vi "MGI Save & Restore Settings.vi"(6 "Section Name (\"Settings\")":string="Settings", 7 "Allow Restore in Development Environment (F)":bool, 8 "Error In":errorcluster, 9 "Command (Restore)":T6, 10 "Path":path, 11 "VI Reference In (Caller)":refnum<vi>) -> (0 "Error Out":errorcluster, 3 "VI Reference Out":refnum<vi>)   [LabVIEW 2016]
doc: "Saves or Restores the settings associated with a VI, including panel bounds, listbox column widths, and graph/chart plots. The settings are saved in an ini file at the specified path. For table style controls, only the columns with headers are saved.\n\nAuthored by Shawn Walpole\nsupport@mooregoodideas.com\nwww.mooregoodideas.com\n\nCopyright (c) 2010, Moore Good Ideas, Inc.\n\nAll rights reserved.\n\nRedistribution and use in source and binary forms, with or without modification, are permitted provided that the following conditions are met:\n\n * Redistributions of source code must retain the above copyright notice, this list of conditions and the following disclaimer.\n * Redistributions in binary form must reproduce the above copyright notice, this list of conditions and the following disclaimer in the documentation and/or other materials provided with the distribution.\n * Neither the name of Moore Good Ideas, Inc. nor the names of its contributors may be used to endorse or promote products derived from this software without specific prior written permission.\n\nTHIS SOFTWARE IS PROVIDED BY THE COPYRIGHT HOLDERS AND CONTRIBUTORS \"AS IS\" AND ANY EXPRESS OR IMPLIED WARRANTIES, INCLUDING, BUT NOT LIMITED TO, THE IMPLIED WARRANTIES OF MERCHANTABILITY AND FITNESS FOR A PARTICULAR PURPOSE ARE DISCLAIMED. IN NO EVENT SHALL THE COPYRIGHT OWNER OR CONTRIBUTORS BE LIABLE FOR ANY DIRECT, INDIRECT, INCIDENTAL, SPECIAL, EXEMPLARY, OR CONSEQUENTIAL DAMAGES (INCLUDING, BUT NOT LIMITED TO, PROCUREMENT OF SUBSTITUTE GOODS OR SERVICES; LOSS OF USE, DATA, OR PROFITS; OR BUSINESS INTERRUPTION) HOWEVER CAUSED AND ON ANY THEORY OF LIABILITY, WHETHER IN CONTRACT, STRICT LIABILITY, OR TORT (INCLUDING NEGLIGENCE OR OTHERWISE) ARISING IN ANY WAY OUT OF THE USE OF THIS SOFTWARE, EVEN IF ADVISED OF THE POSSIBILITY OF SUCH DAMAGE."
uses:
  <userlib>/_MGI/Application Control/MGI Save & Restore Settings/MGI SRS Command Enum.ctl
  <userlib>/_MGI/Application Control/MGI Save & Restore Settings/MGI SRS Graph Setting Cluster.ctl
  <userlib>/_MGI/Application Control/MGI Save & Restore Settings/MGI SRS Graph Plot Cluster.ctl
  <userlib>/_MGI/Application Control/MGI Save & Restore Settings/MGI SRS Graph Cursor Cluster.ctl
  <userlib>/_MGI/Application Control/MGI Save & Restore Settings/MGI SRS MCLB Setting Cluster.ctl
  <userlib>/_MGI/Application Control/MGI Save Restore Settings/Save Restore Settings.lvclass
  <userlib>/_MGI/Application Control/MGI VI Reference/MGI Caller's VI Reference.vi
panel:
  in  "Save Restore Settings in":refnum<class "Save Restore Settings.lvclass">
  in  "Empty":cluster{string, refnum<vi>}[](array[cluster])
  in  "Graph":T1
  in  "MCLB":T4
  in  "Graph":T1
  in  "MCLB":T4
  in  "Empty":cluster{string, refnum<vi>}[](array[cluster])
  in  "Settings":T5
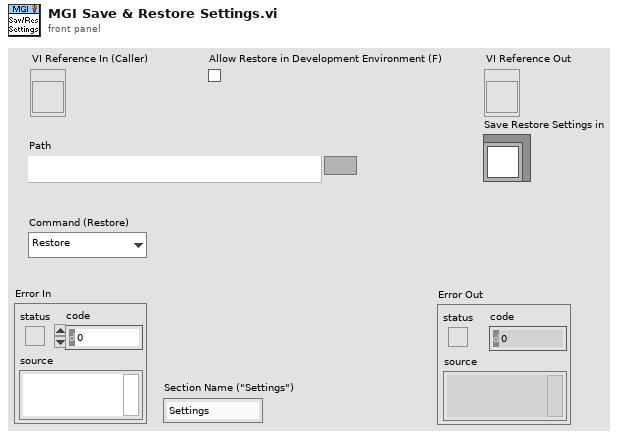
[diagram p1: front panel]
types:
  T1 = typedef "MGI SRS Graph Setting Cluster.ctl" = cluster{"Plot":T2[], "Cursors":T3[], "Cursor Legend?":bool, "Plot Legend?":bool}
  T2 = typedef "MGI SRS Graph Plot Cluster.ctl" = cluster{"Plot Name":string, "Plot Color":u32, "Plot Interpolation":u8, "Point Style":u8, "Line Style":u8, "Fill/Pt. Color":u32, "Line Width":u8, "Bar Plot Style":u8, "Fill To":i16, "XScaleIdx":u32, "YScaleIdx":u32, "Visible?":bool, "Plot Info":cluster{"Plot Color":u32, "Plot Interpolation":u8, "Point Style":u8, "Line Style":u8, "Fill/Pt. Color":u32, "Line Width":u8, "Bar Plot Style":u8, "Fill To":i16}, "Label Style":u8, "Transition Type":u8, "TransitionLocation":u8, "DigitalLineStyle":u8}
  T3 = typedef "MGI SRS Graph Cursor Cluster.ctl" = cluster{"Cursor Name":string, "Cursor Color":u32, "Cursor Style":u8, "Cursor Point Style":u8, "Cursor Name Visible":bool, "Allow Drag":bool, "Cursor Plot":i32, "Cursor Index":i32, "Cursor Position":cluster{"Cursor X":dbl, "Cursor Y":dbl}, "Cursor X":dbl, "Cursor Y":dbl, "Visible":bool, "LineStyle":u8, "LineWidth":u8, "CursorMode":u32, "XScale":u32, "YScale":u32, "WatchPlots":i32[], "WatchAllPlots":bool, "PlotArea":i32, "Label Offset":cluster{"X":dbl, "Y":dbl}}
  T4 = typedef "MGI SRS MCLB Setting Cluster.ctl" = cluster{"Col Widths":i32[]}
  T5 = cluster{"PanelBnds":cluster{"Left":i16, "Top":i16, "Right":i16, "Bottom":i16}, "Splitter Pos":i32[], "Graph Names":string[], "Graph Settings":T1[], "MCLB or Table Names":string[], "MCLB Info":T4[]}
  T6 = typedef "MGI SRS Command Enum.ctl" = enum16{"Restore", "Save"}
  T7 = cluster{"Left":i16, "Top":i16, "Right":i16, "Bottom":i16}
  T8 = typedef "LVRectTypeDef.ctl" = cluster{"Left":i16, "Top":i16, "Right":i16, "Bottom":i16}
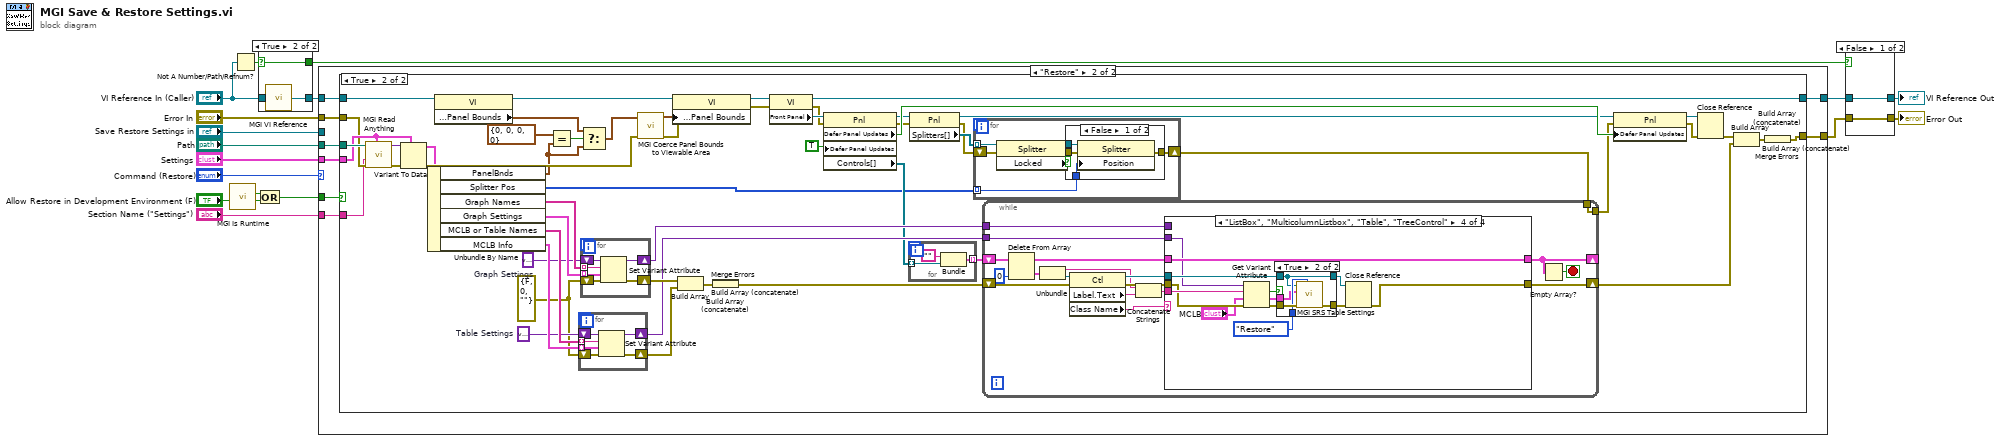
[diagram p0: block diagram]
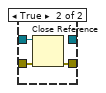
[diagram p2: hidden frame]
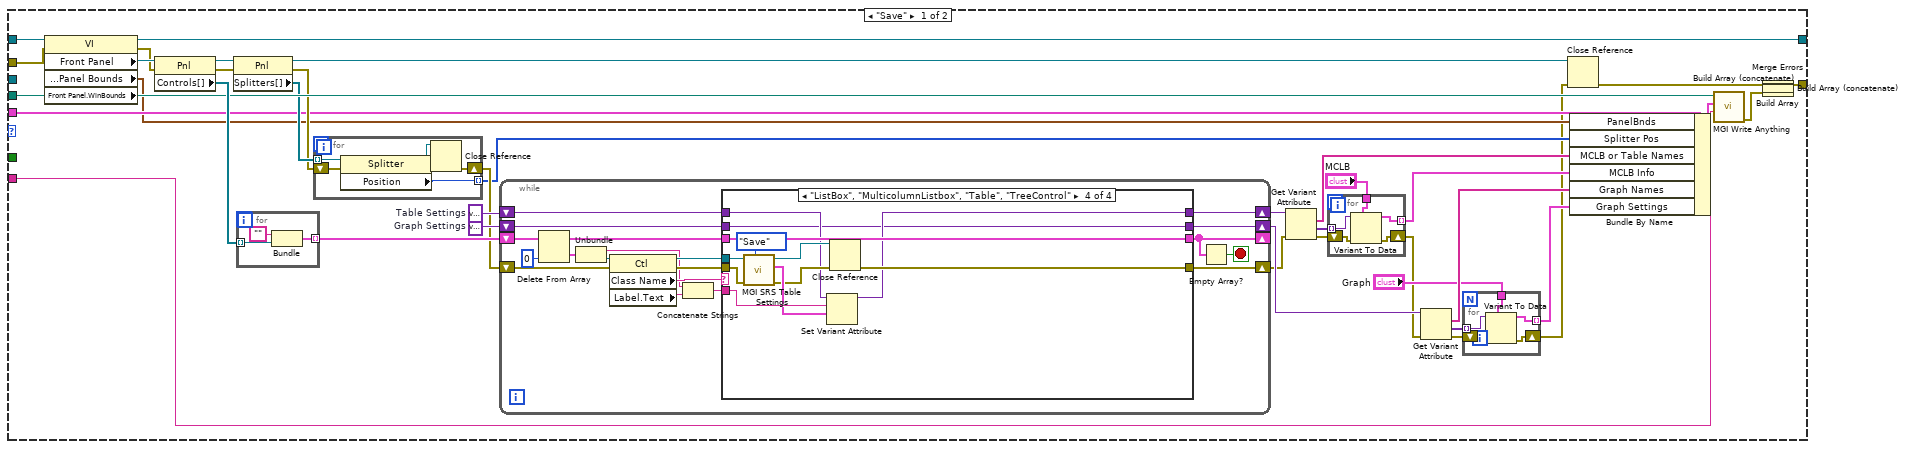
[diagram p3: hidden frame]
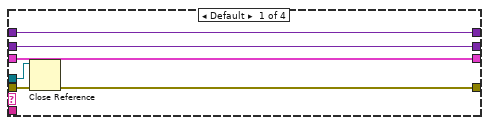
[diagram p4: hidden frame]
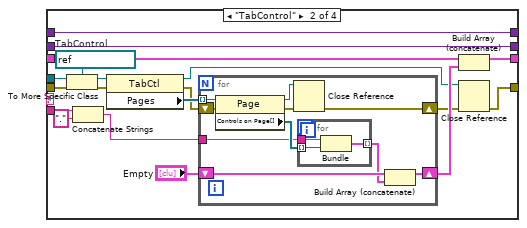
[diagram p5: hidden frame]
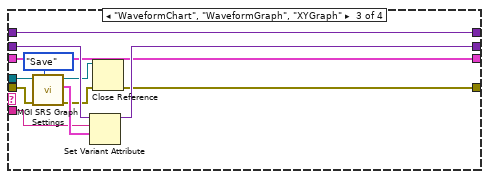
[diagram p6: hidden frame]
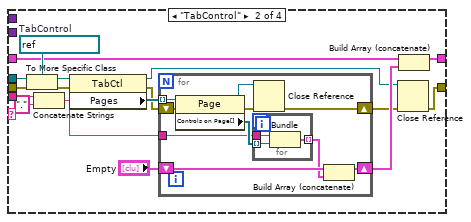
[diagram p10: hidden frame]
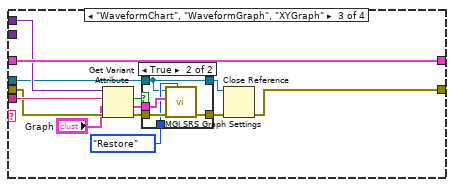
[diagram p11: hidden frame]
diagram:
  n1 = call <userlib>:"MGI Is Runtime.vi"() -> ("Run Time System?"=w4:bool)  [unwired: 7 in]
  n2 = Not A Number/Path/Refnum?(number/path/refnum="VI Reference In (Caller)") -> (NaN/Path/Refnum?=w7:bool)
  n3 = case shown="True" w7 {
    selector: w7 -> [_ w19]
    tunnel: [w18 w20] -> w13
    tunnel: "VI Reference In (Caller)" -> [w18 _]
    tunnel: [_ w19] -> w14
    frame False {
    }
    frame True {
      n4 = call-poly <userlib>:"MGI VI Reference.vi"() -> ("Caller's VI Reference"=w20:refnum<vi>)  [unwired: 1 in]
    }
  }
  n5 = Compound Arithmetic op=OR(w4, "Allow Restore in Development Environment (F)") -> (w3:bool)
  n6 = case shown="\"Restore\"" "Command (Restore)" {
    tunnel: "Path" -> [w43 w167]
    tunnel: [w54 w168] -> w15
    tunnel: "Settings" -> [w32 w166]
    tunnel: w13 -> [w42 w165]
    tunnel: "Error In" -> [w36 w164]
    tunnel: [w25 w163] -> w8
    tunnel: w3 -> [_ w162]
    tunnel: "Section Name (\"Settings\")" -> [w21 w161]
    tunnel: "Save Restore Settings in" -> [_ _]
    frame "Save" {
      w58 = variant  # Graph Settings
      w59 = variant  # Table Settings
      n7 = property class="VI" props=["Front Panel", "Front Panel Window:Panel Bounds", "Front Panel.WinBounds"](reference=w42, error in=w36) -> (reference out=w54:refnum<vi>, error out=w61:errorcluster, "Front Panel"=w62:refnum<vi>, "Front Panel Window:Panel Bounds"=w31:T8)  [unwired: 1 out]
      n8 = property class="Pnl"(reference=w62, error in=w61) -> (reference out=w41:refnum<vi>, error out=w39:errorcluster, "Controls[]"=w60:refnum<vi>[])
      n9 = property class="Pnl"(reference=w41, error in=w39) -> (reference out=w40:refnum<vi>, error out=w37:errorcluster, "Splitters[]"=w38:refnum<vi>[])
      n10 = for {
        tunnel: w60 -> [w81] mode=indexing
        tunnel: [w80] -> w44 mode=indexing
        n11 = Bundle("", w81) -> (w80:cluster{string, refnum<vi>})  [unwired: 1 in]
      }
      n12 = for {
        tunnel: w38 -> [w67] mode=indexing
        tunnel: [w66] -> w30 mode=indexing
        shift-right: [w63] -> w35
        shift-left: w37 -> [w68]
        n13 = property class="Splitter"(reference=w67, error in=w68) -> (reference out=w65:refnum<vi>, error out=w64:errorcluster, "Position"=w66:i32)
        n14 = Close Reference(reference=w65, error in (no error)=w64) -> (error out=w63:errorcluster)
      }
      n15 = while {
        shift-right: [w94] -> w57
        shift-left: w58 -> [w96]
        shift-right: [w95] -> w56
        shift-left: w59 -> [w97]
        shift-right: [w83] -> _
        shift-left: w44 -> [w100]
        shift-right: [w84] -> w29
        shift-left: w35 -> [w87]
        stop <- w82 stop-if-true
        n16 = Delete From Array(array=w100, index=0) -> (deleted portion=w99:cluster{string, refnum<vi>}, array with subset deleted=w98:cluster{string, refnum<vi>}[])  [unwired: 1 in]
        n17 = Unbundle(w99) -> (w85:string, w86:refnum<vi>)
        n18 = property class="Ctl"(reference=w86, error in=w87) -> (reference out=w92:refnum<vi>, error out=w93:errorcluster, "Class Name"=w91:string, "Label.Text"=w90:string)
        n19 = Concatenate Strings(w85, w90) -> (w89:string)
        n20 = case shown="\"ListBox\", \"MulticolumnListbox\", \"Table\", \"TreeControl\"" w91 {
          tunnel: w93 -> [w102 w123 w139 w154]
          tunnel: w98 -> [w106 w115 w144 w160]
          tunnel: w97 -> [w105 w125 w145 w152]
          tunnel: w96 -> [w104 w124 w149 w150]
          tunnel: w89 -> [_ w116 w141 w158]
          tunnel: [w105 w125 w145 w151] -> w95
          tunnel: [w104 w124 w146 w150] -> w94
          tunnel: w92 -> [w103 w122 w140 w157]
          tunnel: [w106 w113 w144 w160] -> w83
          tunnel: [w101 w110 w143 w159] -> w84
          frame Default {
            n21 = Close Reference(reference=w103, error in (no error)=w102) -> (error out=w101:errorcluster)
          }
          frame "TabControl" {
            w121 = refnum<vi> refnum  # TabControl
            n22 = To More Specific Class(target class=w121, reference=w122, error in=w123) -> (specific class reference=w119:refnum<vi>, error out=w120:errorcluster)
            n23 = Concatenate Strings(w116, ".") -> (w108:string)
            n24 = property class="TabCtl"(reference=w119, error in=w120) -> (reference out=w109:refnum<vi>, error out=w117:errorcluster, "Pages"=w118:refnum<vi>[])
            n25 = for {
              tunnel: w118 -> [w135] mode=indexing
              shift-right: [w131] -> w111
              shift-left: w117 -> [w134]
              shift-right: [w127] -> w114
              shift-left: "Empty" -> [w129]
              tunnel: w108 -> [w126]
              n26 = property class="Page"(reference=w135, error in=w134) -> (reference out=w132:refnum<vi>, error out=w133:errorcluster, "Controls on Page[]"=w130:refnum<vi>[])
              n27 = Close Reference(reference=w132, error in (no error)=w133) -> (error out=w131:errorcluster)
              n28 = for {
                tunnel: w130 -> [w138] mode=indexing
                tunnel: [w137] -> w128 mode=indexing
                tunnel: w126 -> [w136]
                n29 = Bundle(w136, w138) -> (w137:cluster{string, refnum<vi>})  [unwired: 1 in]
              }
              n30 = Build Array (concatenate)(w129, w128) -> (w127:cluster{string, refnum<vi>}[])
            }
            n31 = Build Array (concatenate)(w115, w114) -> (w113:cluster{string, refnum<vi>}[])
            n32 = Close Reference(reference=w109, error in (no error)=w111) -> (error out=w110:errorcluster)
          }
          frame "WaveformChart", "WaveformGraph", "XYGraph" {
            n33 = call <userlib>:"MGI SRS Graph Settings.vi"("Command"=MGI_SRS_Command_Enum."Save", "Error In"=w139, "Graph/Chart Ref"=w140) -> ("Error Out"=w142:errorcluster, "Graph Info Out"=w147:T1)  [unwired: 7 in]
            n34 = Set Variant Attribute(Variant=w149, name=w141, value=w147) -> (Variant out=w146:variant)  [unwired: 1 in, 2 out]
            n35 = Close Reference(reference=w140, error in (no error)=w142) -> (error out=w143:errorcluster)
          }
          frame "ListBox", "MulticolumnListbox", "Table", "TreeControl" {
            n36 = call <userlib>:"MGI SRS Table Settings.vi"("Command"=MGI_SRS_Command_Enum."Save", "Error In"=w154, "Graph/Chart Ref"=w157) -> ("Error Out"=w153:errorcluster, "MCLB Info Out"=w155:T4)  [unwired: 7 in]
            n37 = Set Variant Attribute(Variant=w152, name=w158, value=w155) -> (Variant out=w151:variant)  [unwired: 1 in, 2 out]
            n38 = Close Reference(reference=w157, error in (no error)=w153) -> (error out=w159:errorcluster)
          }
        }
        n39 = Empty Array?(array=w83) -> (empty?=w82:bool)
      }
      n40 = Get Variant Attribute(Variant=w56, error in=w29) -> (names=w51:string[], values=w52:variant[], error out=w53:errorcluster)  [unwired: 2 in, 1 out]
      n41 = for {
        shift-right: [w77] -> w28
        shift-left: w53 -> [w78]
        tunnel: w52 -> [w76] mode=indexing
        tunnel: "MCLB" -> [w75]
        tunnel: [w74] -> w50 mode=indexing
        n42 = Variant To Data(error in=w78, type=w75, Variant=w76) -> (data=w74:T4, error out=w77:errorcluster)
      }
      n43 = Get Variant Attribute(Variant=w57, error in=w28) -> (names=w47:string[], values=w46:variant[], error out=w49:errorcluster)  [unwired: 2 in, 1 out]
      n44 = for {
        shift-right: [w72] -> w27
        shift-left: w49 -> [w73]
        tunnel: w46 -> [w71] mode=indexing
        tunnel: "Graph" -> [w70]
        tunnel: [w69] -> w48 mode=indexing
        n45 = Variant To Data(error in=w73, type=w70, Variant=w71) -> (data=w69:T1, error out=w72:errorcluster)
      }
      n46 = Close Reference(reference=w40, error in (no error)=w27) -> (error out=w26:errorcluster)
      n47 = Bundle By Name(cluster=w32, "PanelBnds"=w31, "Splitter Pos"=w30, "MCLB or Table Names"=w51, "MCLB Info"=w50, "Graph Names"=w47, "Graph Settings"=w48) -> (w55:T5)
      n48 = call <userlib>:"MGI Write Anything.vi"("Section Name (Name of \"Anything\")"=w21, "Anything"=w55, "Path (dialog)"=w43) -> ("Error Out"=w45:errorcluster)  [unwired: 6 in, 2 out]
      n49 = Build Array(w26, w45) -> (w24:errorcluster[])
      n50 = Build Array (concatenate)(w24) -> (w23:errorcluster[])
      n51 = Build Array (concatenate)(w23) -> (w22:errorcluster[])
      n52 = Merge Errors(w22) -> (w25:errorcluster)
    }
    frame "Restore" {
      n53 = case shown="True" w162 {
        tunnel: [w170 w225] -> w168
        tunnel: w167 -> [_ w221]
        tunnel: w166 -> [_ w220]
        tunnel: w165 -> [w170 w183]
        tunnel: w164 -> [w169 w201]
        tunnel: [w169 w190] -> w163
        tunnel: w161 -> [_ w171]
        frame False {
        }
        frame True {
          w204 = errorcluster {"status"=FALSE, "code"=0, "source"=""} ("error out")
          w210 = variant  # Table Settings
          w211 = variant  # Graph Settings
          n54 = call <userlib>:"MGI Read Anything.vi"("Type of Anything"=w220, "Error In"=w201, "Section Name (Name of \"Type of Anything\")"=w171, "Path (dialog)"=w221) -> ("Error Out"=w223:errorcluster, "Anything"=w222:variant)  [unwired: 4 in, 2 out]
          n55 = Variant To Data(error in=w223, type=w220, Variant=w222) -> (data=w206:T5, error out=w218:errorcluster)
          n56 = Unbundle By Name(w206) -> ("PanelBnds"=w178:T7, "Splitter Pos"=w196:i32[], "Graph Names"=w215:string[], "Graph Settings"=w214:T1[], "MCLB or Table Names"=w213:string[], "MCLB Info"=w212:T4[])
          n57 = property class="VI"(reference=w183) -> (reference out=w182:refnum<vi>, "Front Panel Window:Panel Bounds"=w176:T8)  [unwired: 1 in, 1 out]
          n58 = Equal?(x=T7 {"Left"=0, "Top"=0, "Right"=0, "Bottom"=0} ("PanelBnds"), y=w178) -> (x = y?=w179:bool)
          n59 = for {
            shift-right: [w245] -> w207
            shift-left: w204 -> [w244]
            tunnel: w213 -> [w243] mode=indexing
            shift-right: [w242] -> w202
            shift-left: w210 -> [w241]
            tunnel: w212 -> [w240] mode=indexing
            n60 = Set Variant Attribute(Variant=w241, name=w243, value=w240, error in=w244) -> (Variant out=w242:variant, error out=w245:errorcluster)  [unwired: 1 out]
          }
          n61 = Select(t=w176, s=w179, f=w178) -> (s? t:f=w177:T8)
          n62 = for {
            shift-right: [w251] -> w208
            shift-left: w204 -> [w250]
            tunnel: w215 -> [w249] mode=indexing
            shift-right: [w248] -> w203
            shift-left: w211 -> [w247]
            tunnel: w214 -> [w246] mode=indexing
            n63 = Set Variant Attribute(Variant=w247, name=w249, value=w246, error in=w250) -> (Variant out=w248:variant, error out=w251:errorcluster)  [unwired: 1 out]
          }
          n64 = call <userlib>:"MGI Coerce Panel Bounds to Viewable Area.vi"("Error In"=w218, "Panel Bounds In"=w177) -> ("Error Out"=w181:errorcluster, "Panel Bounds Out"=w180:T7)  [unwired: 8 in]
          n65 = property class="VI"(reference=w182, error in=w181, "Front Panel Window:Panel Bounds"=w180) -> (reference out=w216:refnum<vi>, error out=w217:errorcluster)
          n66 = Build Array(w208, w207) -> (w184:errorcluster[])
          n67 = Build Array (concatenate)(w184) -> (w174:errorcluster[])
          n68 = Build Array (concatenate)(w174) -> (w172:errorcluster[])
          n69 = Merge Errors(w172) -> (w209:errorcluster)
          n70 = property class="VI"(reference=w216, error in=w217) -> (reference out=w225:refnum<vi>, error out=w226:errorcluster, "Front Panel"=w227:refnum<vi>)
          n71 = property class="Pnl"(reference=w227, error in=w226, "Defer Panel Updates"=TRUE) -> (reference out=w195:refnum<vi>, error out=w187:errorcluster, "Defer Panel Updates"=w205:bool, "Controls[]"=w198:refnum<vi>[])
          n72 = for {
            tunnel: w198 -> [w253] mode=indexing
            tunnel: [w254] -> w197 mode=indexing
            n73 = Bundle("", w253) -> (w254:cluster{string, refnum<vi>})  [unwired: 1 in]
          }
          n74 = property class="Pnl"(reference=w195, error in=w187) -> (reference out=w194:refnum<vi>, error out=w199:errorcluster, "Splitters[]"=w200:refnum<vi>[])
          n75 = for {
            shift-right: [w230] -> w186
            shift-left: w199 -> [w234]
            tunnel: w200 -> [w233] mode=indexing
            tunnel: w196 -> [w228] mode=indexing
            n76 = property class="Splitter"(reference=w233, error in=w234) -> (reference out=w231:refnum<vi>, error out=w232:errorcluster, "Locked"=w229:bool)
            n77 = case shown="False" w229 {
              tunnel: w232 -> [w238 w239]
              tunnel: w231 -> [w237 _]
              tunnel: [w236 w239] -> w230
              tunnel: w228 -> [w235 _]
              frame False {
                n78 = property class="Splitter"(reference=w237, error in=w238, "Position"=w235) -> (error out=w236:errorcluster)  [unwired: 1 out]
              }
              frame True {
              }
            }
          }
          n79 = while {
            shift-right: [w257] -> _
            shift-left: w197 -> [w272]
            shift-right: [w258] -> w189
            shift-left: w209 -> [w261]
            tunnel: w203 -> [w267]
            tunnel: w202 -> [w266]
            tunnel: [w255] -> w188
            tunnel: w186 -> [w255]
            stop <- w256 stop-if-true
            n80 = Delete From Array(array=w272, index=0) -> (deleted portion=w270:cluster{string, refnum<vi>}, array with subset deleted=w269:cluster{string, refnum<vi>}[])  [unwired: 1 in]
            n81 = Unbundle(w270) -> (w259:string, w260:refnum<vi>)
            n82 = property class="Ctl"(reference=w260, error in=w261) -> (reference out=w265:refnum<vi>, error out=w264:errorcluster, "Label.Text"=w262:string, "Class Name"=w268:string)
            n83 = Concatenate Strings(w259, w262) -> (w263:string)
            n84 = case shown="\"ListBox\", \"MulticolumnListbox\", \"Table\", \"TreeControl\"" w268 {
              tunnel: w264 -> [w273 w291 w311 w332]
              tunnel: w269 -> [w274 w282 w317 w337]
              tunnel: w267 -> [_ _ w314 _]
              tunnel: w266 -> [_ _ _ w325]
              tunnel: w263 -> [_ w284 w313 w334]
              tunnel: w265 -> [_ w290 w312 w333]
              tunnel: [w274 w280 w317 w337] -> w257
              tunnel: [w273 w275 w308 w329] -> w258
              frame Default {
              }
              frame "TabControl" {
                w289 = refnum<vi> refnum  # TabControl
                n85 = To More Specific Class(target class=w289, reference=w290, error in=w291) -> (specific class reference=w287:refnum<vi>, error out=w288:errorcluster)
                n86 = Concatenate Strings(w284, ".") -> (w283:string)
                n87 = property class="TabCtl"(reference=w287, error in=w288) -> (reference out=w278:refnum<vi>, error out=w285:errorcluster, "Pages"=w286:refnum<vi>[])
                n88 = for {
                  tunnel: w286 -> [w301] mode=indexing
                  shift-right: [w297] -> w276
                  shift-left: w285 -> [w300]
                  tunnel: w283 -> [w292]
                  shift-right: [w293] -> w281
                  shift-left: "Empty" -> [w295]
                  n89 = property class="Page"(reference=w301, error in=w300) -> (reference out=w298:refnum<vi>, error out=w299:errorcluster, "Controls on Page[]"=w296:refnum<vi>[])
                  n90 = for {
                    tunnel: w296 -> [w304] mode=indexing
                    tunnel: [w303] -> w294 mode=indexing
                    tunnel: w292 -> [w302]
                    n91 = Bundle(w302, w304) -> (w303:cluster{string, refnum<vi>})  [unwired: 1 in]
                  }
                  n92 = Close Reference(reference=w298, error in (no error)=w299) -> (error out=w297:errorcluster)
                  n93 = Build Array (concatenate)(w295, w294) -> (w293:cluster{string, refnum<vi>}[])
                }
                n94 = Close Reference(reference=w278, error in (no error)=w276) -> (error out=w275:errorcluster)
                n95 = Build Array (concatenate)(w282, w281) -> (w280:cluster{string, refnum<vi>}[])
              }
              frame "WaveformChart", "WaveformGraph", "XYGraph" {
                n96 = Get Variant Attribute(Variant=w314, name=w313, default value (empty Variant)="Graph", error in=w311) -> (found=w310:bool, value=w315:T1, error out=w316:errorcluster)  [unwired: 1 out]
                n97 = case shown="True" w310 {
                  tunnel: w312 -> [w318 w320]
                  tunnel: w316 -> [w319 w324]
                  tunnel: w315 -> [_ w323]
                  tunnel: [w319 w322] -> w307
                  tunnel: MGI_SRS_Command_Enum."Restore" -> [_ w321]
                  tunnel: [w318 w320] -> w306
                  frame False {
                  }
                  frame True {
                    n98 = call <userlib>:"MGI SRS Graph Settings.vi"("Command"=w321, "Error In"=w324, "Graph Info In"=w323, "Graph/Chart Ref"=w320) -> ("Error Out"=w322:errorcluster)  [unwired: 6 in, 1 out]
                  }
                }
                n99 = Close Reference(reference=w306, error in (no error)=w307) -> (error out=w308:errorcluster)
              }
              frame "ListBox", "MulticolumnListbox", "Table", "TreeControl" {
                n100 = Get Variant Attribute(Variant=w325, name=w334, default value (empty Variant)="MCLB", error in=w332) -> (found=w331:bool, value=w335:T4, error out=w336:errorcluster)  [unwired: 1 out]
                n101 = case shown="True" w331 {
                  tunnel: w333 -> [w338 w341]
                  tunnel: w336 -> [w339 w344]
                  tunnel: w335 -> [_ w340]
                  tunnel: [w339 w343] -> w328
                  tunnel: MGI_SRS_Command_Enum."Restore" -> [_ w342]
                  tunnel: [w338 w341] -> w327
                  frame False {
                  }
                  frame True {
                    n102 = call <userlib>:"MGI SRS Table Settings.vi"("Command"=w342, "Error In"=w344, "MCLB Info In"=w340, "Graph/Chart Ref"=w341) -> ("Error Out"=w343:errorcluster)  [unwired: 6 in, 1 out]
                  }
                }
                n103 = Close Reference(reference=w327, error in (no error)=w328) -> (error out=w329:errorcluster)
              }
            }
            n104 = Empty Array?(array=w257) -> (empty?=w256:bool)
          }
          n105 = property class="Pnl"(reference=w194, error in=w188, "Defer Panel Updates"=w205) -> (reference out=w192:refnum<vi>, error out=w193:errorcluster)
          n106 = Close Reference(reference=w192, error in (no error)=w193) -> (error out=w191:errorcluster)
          n107 = Build Array(w191, w189) -> (w185:errorcluster[])
          n108 = Build Array (concatenate)(w185) -> (w175:errorcluster[])
          n109 = Build Array (concatenate)(w175) -> (w173:errorcluster[])
          n110 = Merge Errors(w173) -> (w190:errorcluster)
        }
      }
    }
  }
  n111 = case shown="False" w14 {
    tunnel: w8 -> [w346 w349]
    tunnel: [w346 w347] -> w17
    tunnel: w15 -> [w345 w348]
    tunnel: [w345 _] -> w9
    frame False {
    }
    frame True {
      n112 = Close Reference(reference=w348, error in (no error)=w349) -> (error out=w347:errorcluster)
    }
  }
  "Error Out" <- w17
  "VI Reference Out" <- w9
